vi "Cycle.vi"(8 "error in (no error)":errorcluster, 11 "TrialBasedExperiment In":refnum<class "TrialBasedExperiment.lvclass">) -> (0 "error out":errorcluster, 3 "TrialBasedExperiment Out":refnum<class "TrialBasedExperiment.lvclass">)   [LabVIEW 2014, in "AcquisitionCoreObjects.lvlib" / "TrialBasedExperiment.lvclass"]
uses:
  TrialBasedExperiment.lvclass
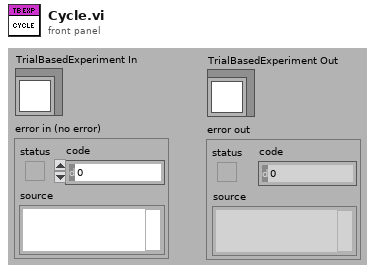
[diagram p1: front panel]
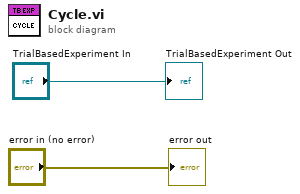
[diagram p0: block diagram]
diagram:
  "TrialBasedExperiment Out" <- "TrialBasedExperiment In"
  "error out" <- "error in (no error)"
